vi "Get Frequency.vi"(8 "error in (no error)":errorcluster, 11 "VISA resource name":refnum<visa-resource-name>) -> (0 "error out":errorcluster, 2 "Frequency":enum16{"50", "60", "400", "800"}(ring)=enum."60", 3 "VISA resource name out":refnum<visa-resource-name>)   [LabVIEW 2020, in "Associated Research 78XX Series.lvlib"]
uses:
  <instrlib>/Associated Research 78XX Series/Associated Research 78XX Series.lvlib
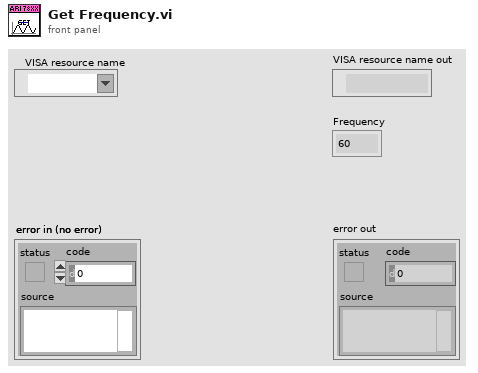
[diagram p1: front panel]
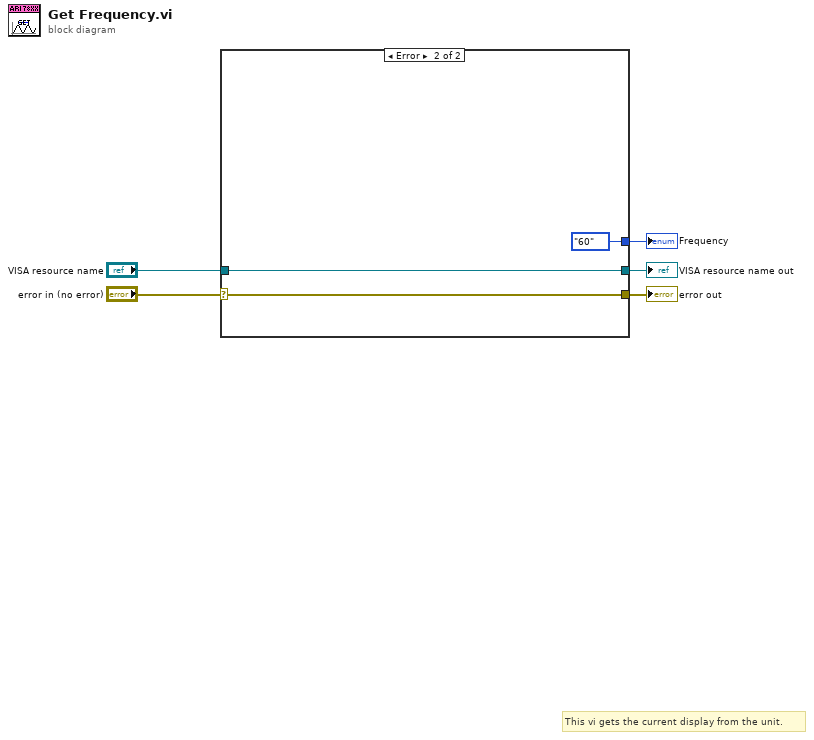
[diagram p0: block diagram]
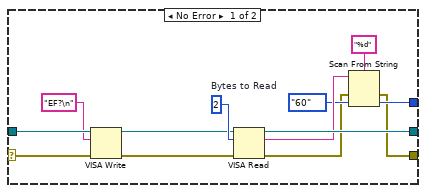
[diagram p2: hidden frame]
diagram:
  # "This vi gets the current display from the unit."
  n1 = case shown="Error" "error in (no error)" {
    selector: "error in (no error)" -> [w18 w21]
    tunnel: [w7 w21] -> w4
    tunnel: [w12 w20] -> w2
    tunnel: "VISA resource name" -> [w17 w20]
    tunnel: [w10 enum16{"50", "60", "400", "800"}."60" ("Frequency")] -> w1
    frame No Error {
      w16 = u32 2  # Bytes to Read
      n2 = VISA Write(VISA resource name=w17, write buffer="EF?\n" ("string (\"\")"), error in (no error)=w18) -> (VISA resource name out=w14:refnum<visa-resource-name>, error out=w13:errorcluster)  [unwired: 1 out]
      n3 = VISA Read(VISA resource name=w14, byte count=w16, error in (no error)=w13) -> (VISA resource name out=w12:refnum<visa-resource-name>, read buffer=w11:string, error out=w8:errorcluster)  [unwired: 1 out]
      n4 = Scan From String(format string="%d", input string=w11, error in=w8, default 1=enum16{"50", "60", "400", "800"}."60" ("Frequency")) -> (error out=w7:errorcluster, output 1=w10:enum16{"50", "60", "400", "800"})  [unwired: 1 in, 2 out]
    }
    frame Error {
    }
  }
  "error out" <- w4
  "VISA resource name out" <- w2
  "Frequency" <- w1
